vi "SR5302 GPIB Write-Read_mod.vi"(0 "VISA session (for class)":refnum<visa-resource-name>, 1 "Write Command String":string, 2 "DC Command":bool, 3 "Curve Length":u16=100 min=1, 5 "error in (no error)":errorcluster) -> (8 "Invalid Command":bool, 9 "Reference Unlock":bool, 10 "Command Parameter error":bool, 11 "ADC Triggered":bool, 12 "Output Data Array":string[](array[string]), 13 "Overload":bool, 14 "VISA session":refnum<visa-resource-name>, 15 "Response 1":string, 16 "Response 2":string, 17 "Response 3":string, 18 "Response 4":string, 19 "error out":errorcluster)   [LabVIEW 2015]
doc: "This VI should be used instead of standard VISA write or write-read constructs since it supports the software handshaking required when using the RS232 interface. It also handles the follwing types if instrument response:-\nSingle response, e.g. to X (output) command\nMultiple responses, e.g. to M (monitor) command\nArray responses, e.g. to DC (dump curve) command. In order to handle these, the VI needs to know that the command is DC and the curve length to dowload.\n\nIt also reports the instrument's status\n\n18/5/05 First Release for LV 7.1"
panel:
  out "Numeric":i32
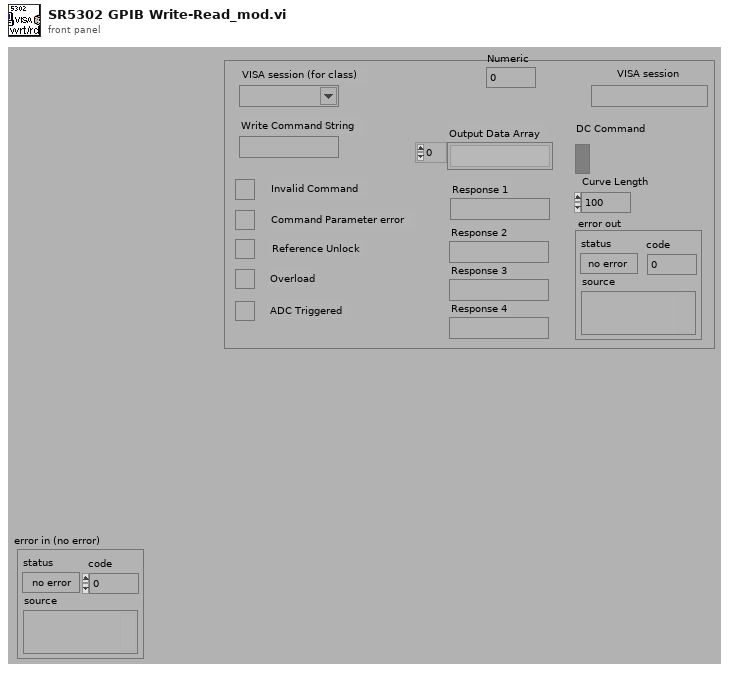
[diagram p1: front panel]
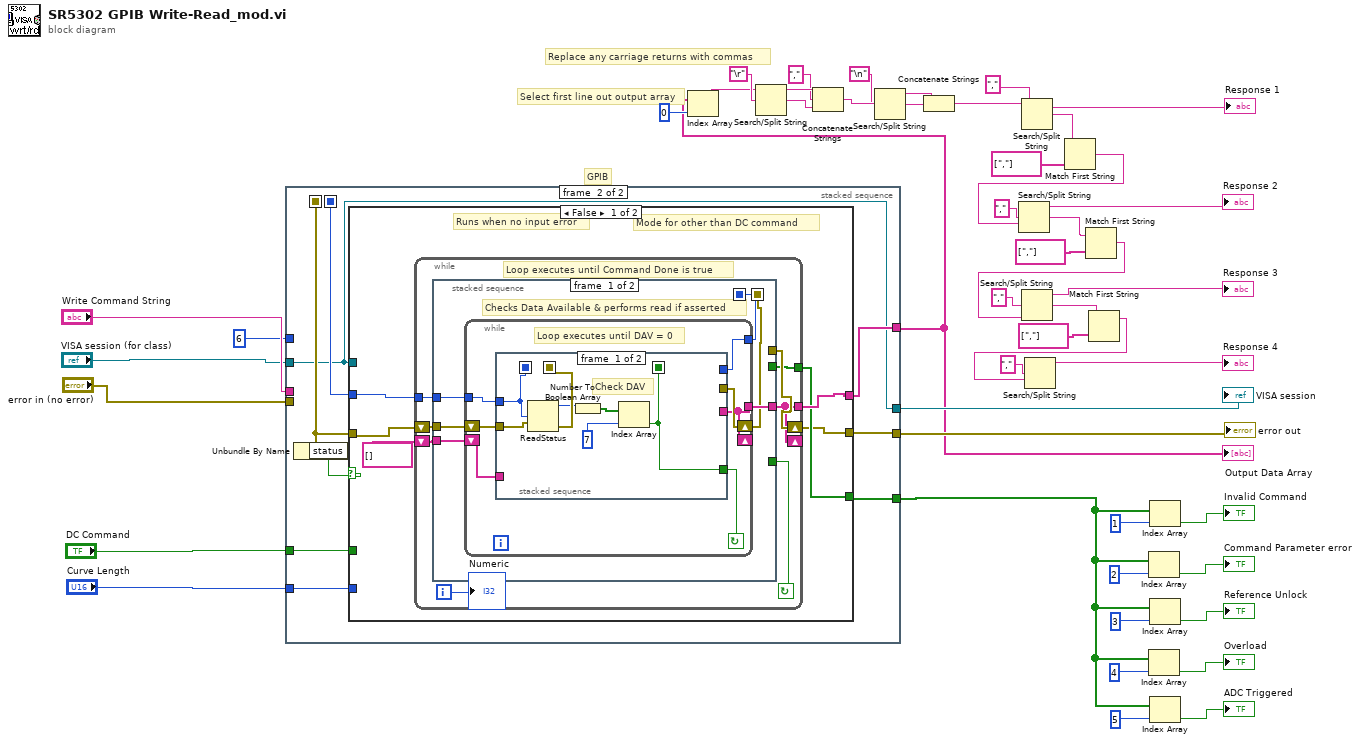
[diagram p0: block diagram]
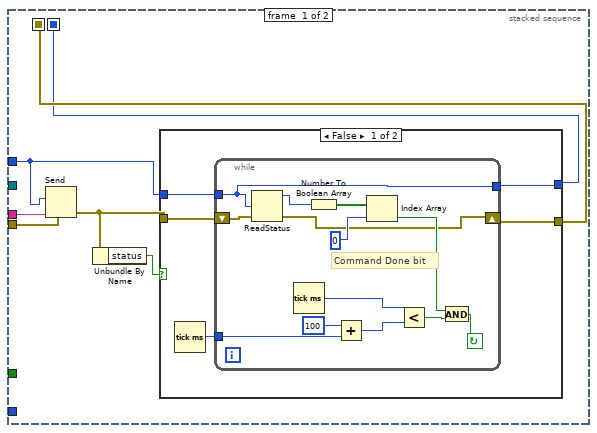
[diagram p2: hidden frame]
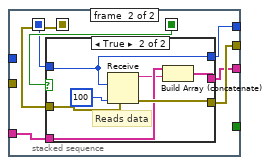
[diagram p4: hidden frame]
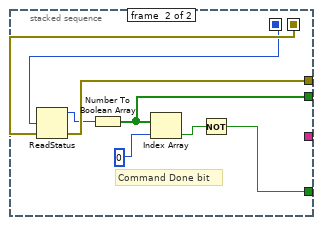
[diagram p6: hidden frame]
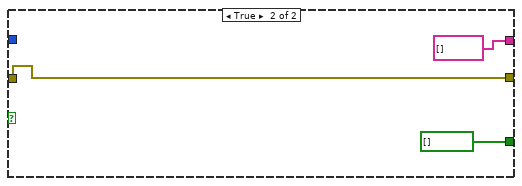
[diagram p7: hidden frame]
diagram:
  # "GPIB"
  # "Select first line out output array"
  # "Replace any carriage returns with commas"
  n1 = stacked-sequence {
    seq-local: [w54 _] -> [_ w80]
    seq-local: [w55 _] -> [_ w79]
    tunnel: [_ w76] -> w47
    tunnel: [_ w84] -> w46
    tunnel: "Write Command String" -> [w50 _]
    tunnel: "VISA session (for class)" -> [_ w76]
    tunnel: "error in (no error)" -> [w51 _]
    tunnel: [_ w83] -> w6
    tunnel: [_ w82] -> w32
    tunnel: "DC Command" -> [_ w78]
    tunnel: "Curve Length" -> [_ w77]
    tunnel: i16 6 ("address") -> [w49 _]
    frame #0 {
      n2 = Send(2:w49, 4:w51, 5:w50) -> (8:w52:errorcluster)  [unwired: 2 in, 2 out]
      n3 = Unbundle By Name(w52) -> ("status"=w53:bool)
      n4 = case shown="False" w53 {
        tunnel: [w60 w74] -> w55
        tunnel: [w59 w75] -> w54
        tunnel: w49 -> [w57 w75]
        tunnel: w52 -> [w56 w74]
        frame False {
          n5 = Tick Count (ms)() -> (millisecond timer value=w58:u32)
          n6 = while {
            tunnel: [w61] -> w59
            tunnel: w57 -> [w61]
            tunnel: w58 -> [w65]
            shift-right: [w63] -> w60
            shift-left: w56 -> [w64]
            stop <- w67 continue-if-true
            # "Command Done bit"
            n7 = ReadStatus(3:w64, 4:w61) -> (0:w63:errorcluster, 2:w62:i16)  [unwired: 1 in, 1 out]
            n8 = Tick Count (ms)() -> (millisecond timer value=w70:u32)
            n9 = Number To Boolean Array(number=w62) -> (Boolean array=w73:bool[])
            n10 = Add(x=u32 100, y=w65) -> (x+y=w69:u32)
            n11 = Index Array(array=w73, index=0) -> (element=w71:bool)
            n12 = Less?(x=w70, y=w69) -> (x < y?=w66:bool)
            n13 = And(x=w71, y=w66) -> (x .and. y?=w67:bool)
          }
        }
        frame True {
        }
      }
    }
    frame #1 {
      n14 = Unbundle By Name(w79) -> ("status"=w81:bool)
      n15 = case shown="False" w81 {
        tunnel: [w90 string[] []] -> w82
        tunnel: [w89 bool[] []] -> w83
        tunnel: w79 -> [w88 w146]
        tunnel: w80 -> [w87 _]
        tunnel: [w86 w146] -> w84
        tunnel: w78 -> [_ _]
        tunnel: w77 -> [_ _]
        tunnel: w76 -> [_ _]
        frame False {
          # "Mode for other than DC command"
          # "Runs when no input error"
          n16 = while {
            shift-left: string[] [] -> [w93]
            shift-right: [w94] -> _
            tunnel: [w94] -> w90
            tunnel: [w92] -> w89
            tunnel: w87 -> [w95]
            shift-right: [w98] -> w86
            shift-left: w88 -> [w96]
            i -> [w91]
            stop <- w97 continue-if-true
            # "Loop executes until Command Done is true"
            n17 = stacked-sequence {
              seq-local: [w102 _] -> [_ w141]
              seq-local: [w99 _] -> [_ w137]
              tunnel: [w104 _] -> w94
              tunnel: w95 -> [w103 _]
              tunnel: [_ w138] -> w97
              tunnel: [_ w140] -> w98
              tunnel: [_ w139] -> w92
              tunnel: w96 -> [w101 _]
              tunnel: w93 -> [w100 _]
              frame #0 {
                # "Checks Data Available & performs read if asserted"
                n18 = while {
                  tunnel: [w106] -> w99
                  shift-left: w100 -> [w107]
                  shift-right: [w108] -> _
                  tunnel: [w108] -> w104
                  tunnel: w103 -> [w111]
                  shift-right: [w109] -> w102
                  shift-left: w101 -> [w110]
                  stop <- w105 continue-if-true
                  # "Loop executes until DAV = 0"
                  n19 = stacked-sequence {
                    seq-local: [w114 _] -> [_ w125]
                    seq-local: [w115 _] -> [_ w124]
                    seq-local: [w113 _] -> [_ w120]
                    tunnel: w111 -> [w113 _]
                    tunnel: [_ w122] -> w108
                    tunnel: w110 -> [w116 _]
                    tunnel: [_ w123] -> w109
                    tunnel: [w114 _] -> w105
                    tunnel: w107 -> [_ w121]
                    tunnel: [_ w119] -> w106
                    frame #0 {
                      # "Check DAV"
                      n20 = ReadStatus(3:w116, 4:w113) -> (0:w115:errorcluster, 2:w112:i16)  [unwired: 1 in, 1 out]
                      n21 = Number To Boolean Array(number=w112) -> (Boolean array=w118:bool[])
                      n22 = Index Array(array=w118, index=7) -> (element=w114:bool)
                    }
                    frame #1 {
                      n23 = case shown="True" w125 {
                        tunnel: w120 -> [w126 w130]
                        tunnel: [w127 w134] -> w122
                        tunnel: w124 -> [w128 w132]
                        tunnel: [w128 w135] -> w123
                        tunnel: w121 -> [w127 w133]
                        tunnel: [w126 w130] -> w119
                        frame False {
                        }
                        frame True {
                          # "Reads data"
                          n24 = Receive(4:w132, 6:100 ("byte count"), 8:w130) -> (0:w135:errorcluster, 3:w129:string)  [unwired: 2 in, 2 out]
                          n25 = Build Array (concatenate)(w133, w129) -> (w134:string[])
                        }
                      }
                    }
                  }
                }
              }
              frame #1 {
                # "Command Done bit"
                n26 = ReadStatus(3:w141, 4:w137) -> (0:w140:errorcluster, 2:w136:i16)  [unwired: 1 in, 1 out]
                n27 = Number To Boolean Array(number=w136) -> (Boolean array=w139:bool[])
                n28 = Index Array(array=w139, index=0) -> (element=w142:bool)
                n29 = Not(x=w142) -> (.not. x?=w138:bool)
              }
            }
            "Numeric" <- w91
          }
        }
        frame True {
        }
      }
    }
  }
  "VISA session" <- w47
  "error out" <- w46
  "Output Data Array" <- w32
  n30 = Index Array(array=w32, index=0) -> (element=w33:string)
  n31 = Search/Split String(string=w33, search string/char (-)="\r" ("search char (-)")) -> (substring before match=w41:string, match + rest of string=w38:string)  [unwired: 1 in, 1 out]
  n32 = Concatenate Strings(w41, "," ("substring before char"), w38) -> (w40:string)
  n33 = Search/Split String(string=w40, search string/char (-)="\n" ("search char (-)")) -> (substring before match=w35:string, match + rest of string=w36:string)  [unwired: 1 in, 1 out]
  n34 = Concatenate Strings(w35, w36) -> (w34:string)
  n35 = Search/Split String(string=w34, search string/char (-)="," ("search char (-)")) -> (substring before match=→"Response 1":string, match + rest of string=w17:string)  [unwired: 1 in, 1 out]
  n36 = Match First String(2:string[] [","] ("string array"), 3:w17) -> (1:w25:string)  [unwired: 1 out]
  n37 = Search/Split String(string=w25, search string/char (-)="," ("search char (-)")) -> (substring before match=→"Response 2":string, match + rest of string=w23:string)  [unwired: 1 in, 1 out]
  n38 = Match First String(2:string[] [","] ("string array"), 3:w23) -> (1:w22:string)  [unwired: 1 out]
  n39 = Search/Split String(string=w22, search string/char (-)="," ("search char (-)")) -> (substring before match=→"Response 3":string, match + rest of string=w28:string)  [unwired: 1 in, 1 out]
  n40 = Match First String(2:string[] [","] ("string array"), 3:w28) -> (1:w19:string)  [unwired: 1 out]
  n41 = Search/Split String(string=w19, search string/char (-)="," ("search char (-)")) -> (substring before match=→"Response 4":string)  [unwired: 1 in, 2 out]
  n42 = Index Array(array=w6, index=2) -> (element=→"Command Parameter error":bool)
  n43 = Index Array(array=w6, index=4) -> (element=→"Overload":bool)
  n44 = Index Array(array=w6, index=1) -> (element=→"Invalid Command":bool)
  n45 = Index Array(array=w6, index=3) -> (element=→"Reference Unlock":bool)
  n46 = Index Array(array=w6, index=5) -> (element=→"ADC Triggered":bool)
